vi "GetSaveRate.vi"(8 "error in (no error)":errorcluster, 11 "FAMM in":refnum<class "FAMM.lvclass">) -> (0 "error out":errorcluster, 2 "Dbase saving period (sec)":dbl, 3 "FAMM out":refnum<class "FAMM.lvclass">)   [LabVIEW 2020, in "FAMM.lvclass"]
doc: "Andre Koelewijn, 2 jan 2021\n\nGet Database Save rate (seconds)"
uses:
  FAMM.lvclass
  FAMM.lvclass/FAMM.ctl
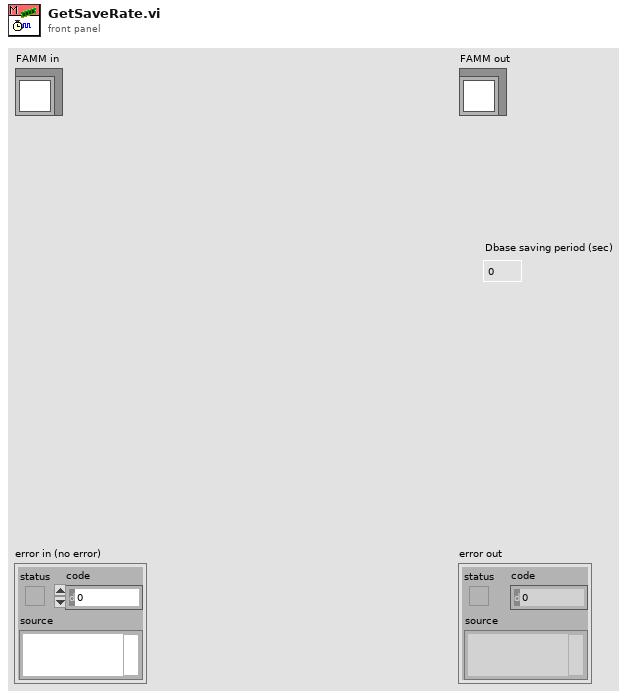
[diagram p1: front panel]
types:
  T1 = typedef "FAMM.lvclass/FAMM-attributes.ctl" = cluster{"FAMM_PAQ_Layers":i32, "FAMM_PAQ_resolution":dbl, "PAQ_TAGs":string[], "WAQ_TAGs":string[], "EAQ_TAGs":string[], "All_TAGs":string[], "PAQtagProps":T2[], "WAQtagProps":T2[], "EAQtagProps":T2[], "DBAL_class":refnum<data-value>, "PAQ_memory":refnum<data-value>[], "PAQupdates":timestamp[], "FAMM_Size":cluster{"other":i32, "1day":i32, "1week":i32}, "DatabaseFileExtention":string, "DatabaseSaveRate":dbl, "Database_path":path}
  T2 = typedef "typedef_com_TagProp.ctl" = cluster{"Description":string, "EngUnits":string, "RangeH":dbl, "RangeL":dbl, "Resolution":i32, "Obsolete":bool, "ChangeDate":timestamp, "ChangeSource":string, "ChangeReason":string, "TagFunc":u32}
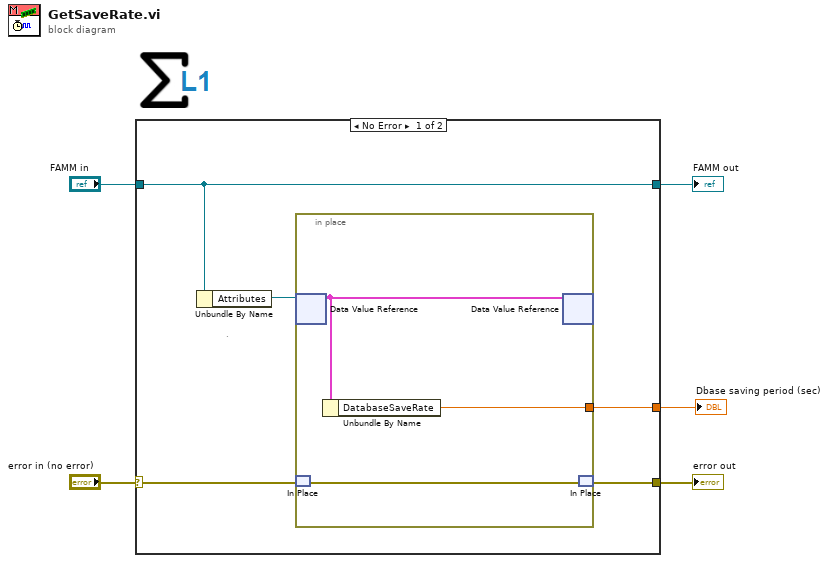
[diagram p0: block diagram]
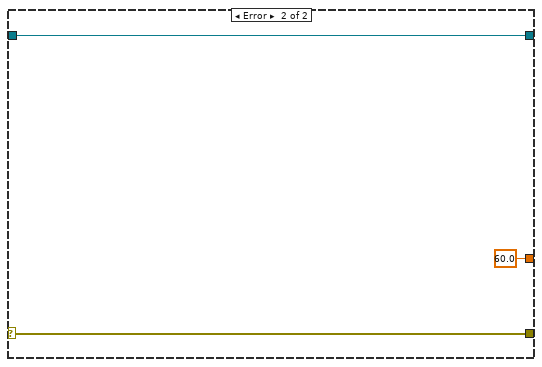
[diagram p2: hidden frame]
diagram:
  n1 = case shown="No Error" "error in (no error)" {
    selector: "error in (no error)" -> [w10 w16]
    tunnel: [w9 w16] -> w4
    tunnel: [w7 w15] -> w2
    tunnel: "FAMM in" -> [w7 w15]
    tunnel: [w6 60.0 ("DatabaseSaveRate")] -> w1
    frame No Error {
      # "`"
      n2 = Unbundle By Name(w7) -> ("Attributes"=w8:refnum<data-value>)
      n3 = in-place {
        in-place-border: [w11] -> w6
        n4 = in-place-dvr #1(w8) -> (w13:T1)  [unwired: 1 out]
        n5 = in-place-match #2(w10) -> (w12:errorcluster)
        n6 = Unbundle By Name(w13) -> ("DatabaseSaveRate"=w11:dbl)
        n7 = in-place-dvr #1(w13) -> ()  [unwired: 2 out]
        n8 = in-place-match #2(w12) -> (w9:errorcluster)
      }
    }
    frame Error {
    }
  }
  "error out" <- w4
  "FAMM out" <- w2
  "Dbase saving period (sec)" <- w1
